vi "SQL指令输入.vi"(8 "error in (no error)":errorcluster, 9 "需要数据？":bool, 10 "SQL query":string, 11 "连接输入":T1) -> (0 "error out":errorcluster, 1 "标签数据存在？":bool, 2 "数据库数据":string[][](array[string]), 3 "连接输出":T1, 4 "标签数据不重复？":bool)   [LabVIEW 2017]
uses:
  <vilib>/addons/database/Connection.llb/Conn ObjectReference.ctl
  <vilib>/addons/database/Connection.llb/Conn Execute.vi
  <vilib>/addons/database/Recordset.llb/Rec Fetch Recordset Data (R).vi
  <vilib>/addons/database/Recordset.llb/Rec Destroy - Connection.vi
  <vilib>/addons/database/NI_Database_API.lvlib
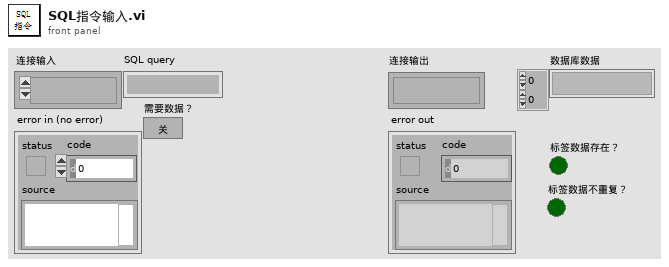
[diagram p1: front panel]
types:
  T1 = typedef "NI_Database_API.lvlib/Conn ObjectReference.ctl" = refnum<k1>
  T2 = typedef "NI_Database_API.lvlib/Rec ObjectReference.ctl" = refnum<k1>
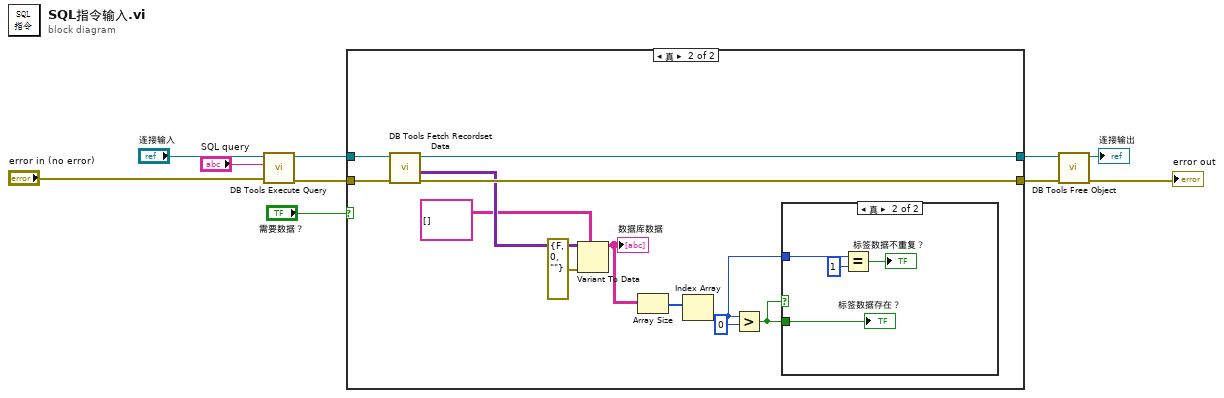
[diagram p0: block diagram]
diagram:
  n1 = call-poly <vilib>:"DB Tools Execute Query.vi"("error in (no error)"="error in (no error)", "SQL query"="SQL query", "connection reference"="连接输入") -> ("error out"=w9:errorcluster, "recordset reference"=w10:T2)  [unwired: 5 in]
  n2 = case shown="真" "需要数据？" {
    tunnel: w10 -> [w12 w24]
    tunnel: w9 -> [w11 w23]
    tunnel: [w12 w22] -> w8
    tunnel: [w11 w21] -> w7
    frame False {
    }
    frame True {
      n3 = call-poly <vilib>:"DB Tools Fetch Recordset Data.vi"("error in (no error)"=w23, "recordset reference"=w24) -> ("error out"=w21:errorcluster, "recordset data"=w19:variant[][], "recordset reference out"=w22:T2)  [unwired: 3 in]
      n4 = Variant To Data(error in=errorcluster {"status"=FALSE, "code"=0, "source"=""} ("错误输入"), type=string[][] [], Variant=w19) -> (data=w17:string[][])  [unwired: 1 out]
      "数据库数据" <- w17
      n5 = Array Size(array=w17) -> (size(s)=w16:i32[])
      n6 = Index Array(array=w16) -> (element=w13:i32)  [unwired: 1 in]
      n7 = Greater?(x=w13, y=0) -> (0:w14:bool)
      n8 = case shown="真" w14 {
        tunnel: w14 -> [_ w28]
        tunnel: w13 -> [_ w27]
        frame False {
        }
        frame True {
          n9 = Equal?(x=w27, y=1) -> (x = y?=→"标签数据不重复？":bool)
          "标签数据存在？" <- w28
        }
      }
    }
  }
  n10 = call-poly <vilib>:"DB Tools Free Object.vi"("error in (no error)"=w7, "recordset reference"=w8) -> ("error out"=→"error out":errorcluster, "connection reference"=→"连接输出":T1)  [unwired: 8 in]
